vi "Constructor.vi"(8 "error in (no error)":errorcluster, 11 "GumballMachine in":refnum<class "GumballMachine.lvclass">) -> (0 "error out":errorcluster, 3 "GumballMachine out":refnum<class "GumballMachine.lvclass">)   [LabVIEW 2013, in "GumballMachine.lvclass"]
uses:
  GumballMachine.lvclass
  SoldOutState.lvclass/SoldOutState.lvclass
  SoldState.lvclass/SoldState.lvclass
  NoCoinState.lvclass/NoCoinState.lvclass
  HasCoinState.lvclass/HasCoinState.lvclass
  GumballMachine.lvclass/GumballMachine.ctl
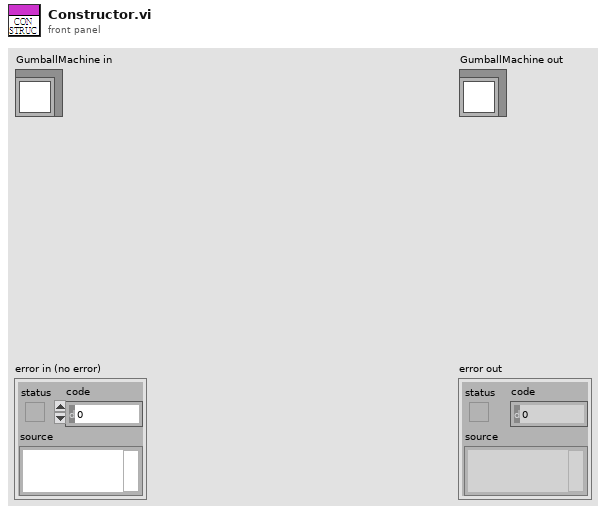
[diagram p1: front panel]
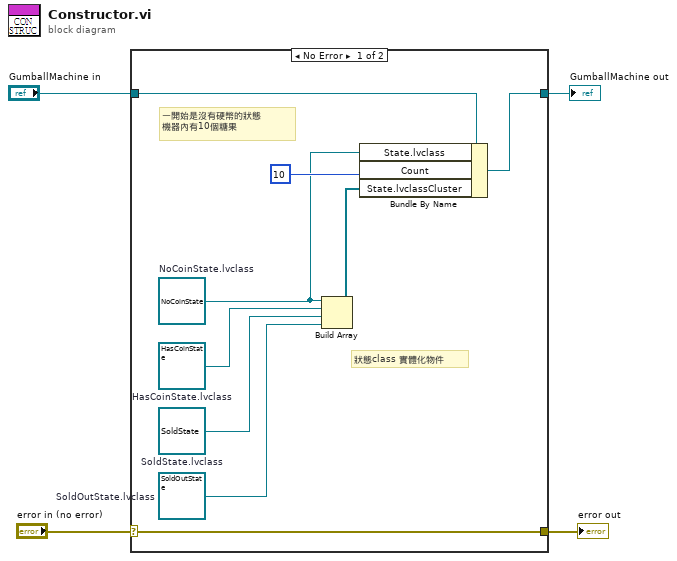
[diagram p0: block diagram]
diagram:
  n1 = case shown="No Error" "error in (no error)" {
    selector: "error in (no error)" -> [w13 w15]
    tunnel: [w13 w15] -> w3
    tunnel: [w11 w14] -> w1
    tunnel: "GumballMachine in" -> [w12 w14]
    frame No Error {
      w8 = refnum<class "HasCoinState.lvclass"> refnum  # HasCoinState.lvclass
      w9 = refnum<class "NoCoinState.lvclass"> refnum  # NoCoinState.lvclass
      w7 = refnum<class "SoldState.lvclass"> refnum  # SoldState.lvclass
      w6 = refnum<class "SoldOutState.lvclass"> refnum  # SoldOutState.lvclass
      # "狀態class 實體化物件"
      # "一開始是沒有硬幣的狀態\n機器內有10個糖果"
      n2 = Build Array(w9, w8, w7, w6) -> (w5:refnum<class "State.lvclass">[])
      n3 = Bundle By Name(cluster=w12, "State.lvclass"=w9, "Count"=10, "State.lvclassCluster"=w5) -> (w11:refnum<class "GumballMachine.lvclass">)
    }
    frame Error {
    }
  }
  "error out" <- w3
  "GumballMachine out" <- w1
